vi "推導公式.vi"(3 "be":i16 min=0, 4 "al":i16 min=0, 5 "移動z":i16 min=0) -> (0 "L3":dbl, 1 "L2":dbl, 2 "L1":dbl)   [LabVIEW 2019]
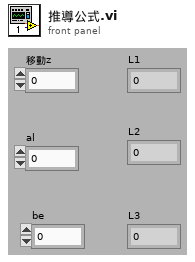
[diagram p1: front panel]
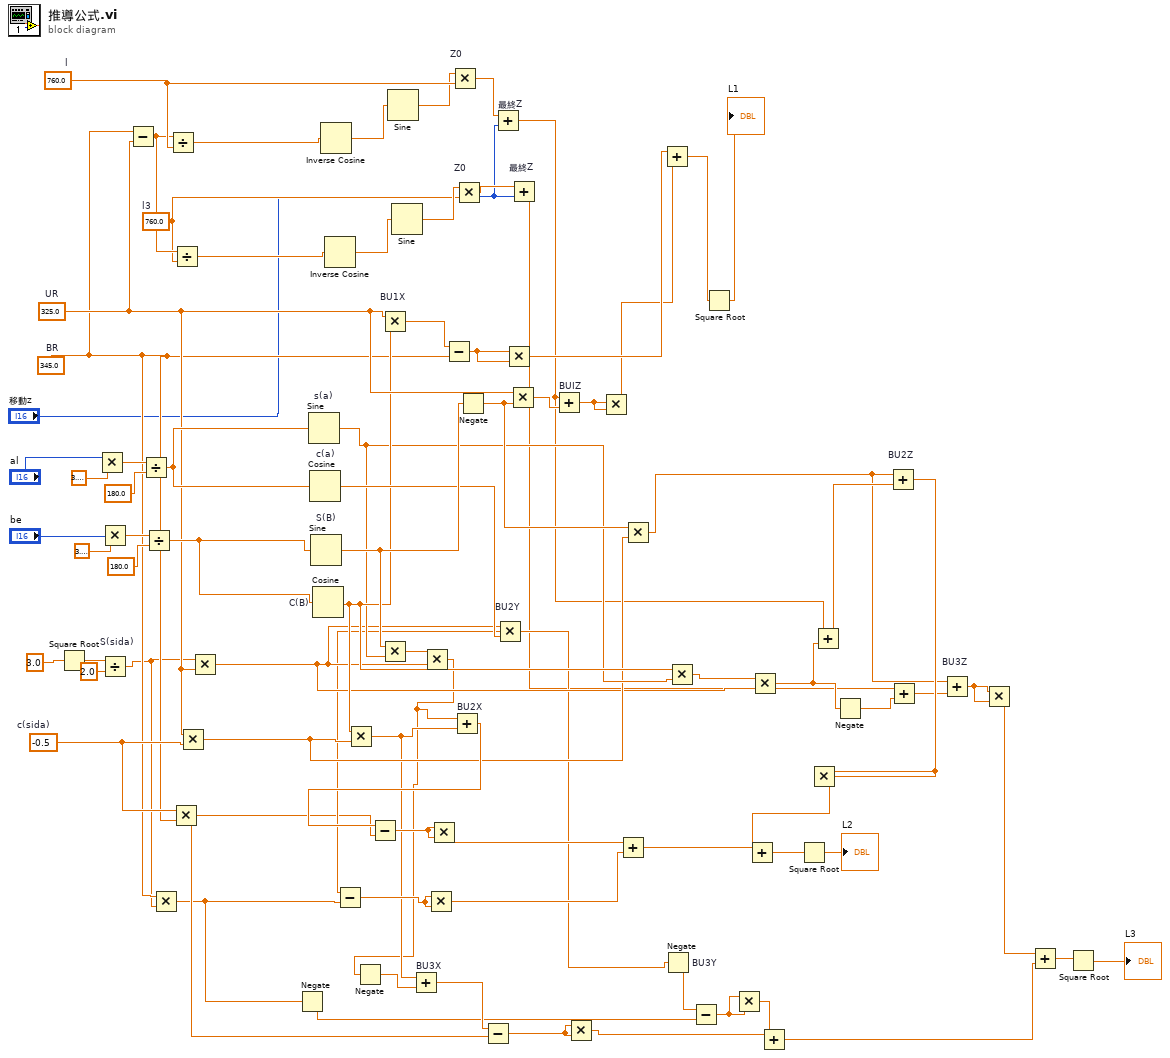
[diagram p0: block diagram]
diagram:
  w4 = 760.0  # l3
  w64 = 760.0  # l
  w29 = 345.0  # BR
  w46 = -0.5  # c(sida)
  w55 = 325.0  # UR
  n1 = Square Root(x=3.0) -> (sqrt(x)=w80:dbl)
  n2 = Multiply(x="al", y=3.141592653589793) -> (x*y=w76:dbl)
  n3 = Multiply(x="be", y=3.141592653589793) -> (x*y=w73:dbl)
  n4 = Divide "S(sida)"(x=w80, y=2.0) -> (x/y=w28:dbl)
  n5 = Subtract(x=w29, y=w55) -> (x-y=w6:dbl)
  n6 = Divide(x=w76, y=180.0) -> (x/y=w70:dbl)
  n7 = Divide(x=w73, y=180.0) -> (x/y=w69:dbl)
  n8 = Multiply(x=w29, y=w28) -> (x*y=w24:dbl)
  n9 = Divide(x=w6, y=w64) -> (x/y=w66:dbl)
  n10 = Multiply(x=w46, y=w29) -> (x*y=w25:dbl)
  n11 = Divide(x=w6, y=w4) -> (x/y=w5:dbl)
  n12 = Multiply(x=w55, y=w46) -> (x*y=w36:dbl)
  n13 = Multiply(x=w28, y=w55) -> (x*y=w34:dbl)
  n14 = Negate(x=w24) -> (-x=w22:dbl)
  n15 = Sine "s(a)"(x=w70) -> (sin(x)=w49:dbl)
  n16 = Cosine "c(a)"(x=w70) -> (cos(x)=w52:dbl)
  n17 = Sine "S(B)"(x=w69) -> (sin(x)=w54:dbl)
  n18 = Cosine "C(B)"(x=w69) -> (cos(x)=w50:dbl)
  n19 = Inverse Cosine(1:w66) -> (0:w65:dbl)
  n20 = Inverse Cosine(1:w5) -> (0:w8:dbl)
  n21 = Multiply(x=w50, y=w36) -> (x*y=w35:dbl)
  n22 = Multiply "BU1X"(x=w55, y=w50) -> (x*y=w68:dbl)
  n23 = Multiply(x=w54, y=w49) -> (x*y=w53:dbl)
  n24 = Sine(x=w65) -> (sin(x)=w63:dbl)
  n25 = Sine(x=w8) -> (sin(x)=w7:dbl)
  n26 = Multiply(x=w53, y=w34) -> (x*y=w32:dbl)
  n27 = Negate(x=w32) -> (-x=w33:dbl)
  n28 = Add "BU3X"(x=w35, y=w33) -> (x+y=w30:dbl)
  n29 = Subtract(x=w68, y=w29) -> (x-y=w67:dbl)
  n30 = Multiply "Z0"(x=w63, y=w64) -> (x*y=w62:dbl)
  n31 = Add "BU2X"(x=w32, y=w35) -> (x+y=w47:dbl)
  n32 = Subtract(x=w47, y=w25) -> (x-y=w45:dbl)
  n33 = Multiply(x=w45, y=w45) -> (x*y=w44:dbl)
  n34 = Multiply "Z0"(x=w7, y=w4) -> (x*y=w3:dbl)
  n35 = Negate(x=w54) -> (-x=w51:dbl)
  n36 = Subtract(x=w30, y=w25) -> (x-y=w27:dbl)
  n37 = Add "最終Z"(x=w62, y="移動z") -> (x+y=w16:dbl)
  n38 = Multiply "BU2Y"(x=w34, y=w52) -> (x*y=w31:dbl)
  n39 = Subtract(x=w31, y=w24) -> (x-y=w43:dbl)
  n40 = Multiply(x=w43, y=w43) -> (x*y=w42:dbl)
  n41 = Multiply(x=w67, y=w67) -> (x*y=w59:dbl)
  n42 = Multiply(x=w55, y=w51) -> (x*y=w61:dbl)
  n43 = Add "最終Z"(x=w3, y="移動z") -> (x+y=w1:dbl)
  n44 = Add "BUIZ"(x=w16, y=w61) -> (x+y=w60:dbl)
  n45 = Multiply(x=w27, y=w27) -> (x*y=w26:dbl)
  n46 = Multiply(x=w60, y=w60) -> (x*y=w58:dbl)
  n47 = Add(x=w44, y=w42) -> (x+y=w41:dbl)
  n48 = Multiply(x=w51, y=w36) -> (x*y=w14:dbl)
  n49 = Add(x=w59, y=w58) -> (x+y=w57:dbl)
  n50 = Negate "BU3Y"(x=w31) -> (-x=w23:dbl)
  n51 = Multiply(x=w50, y=w49) -> (x*y=w48:dbl)
  n52 = Subtract(x=w23, y=w22) -> (x-y=w21:dbl)
  n53 = Square Root(x=w57) -> (sqrt(x)=→"L1":dbl)
  n54 = Multiply(x=w21, y=w21) -> (x*y=w20:dbl)
  n55 = Multiply(x=w48, y=w34) -> (x*y=w18:dbl)
  n56 = Add(x=w26, y=w20) -> (x+y=w12:dbl)
  n57 = Add(x=w16, y=w18) -> (x+y=w19:dbl)
  n58 = Negate(x=w18) -> (-x=w17:dbl)
  n59 = Add "BU2Z"(x=w14, y=w19) -> (x+y=w40:dbl)
  n60 = Multiply(x=w40, y=w40) -> (x*y=w39:dbl)
  n61 = Add(x=w41, y=w39) -> (x+y=w38:dbl)
  n62 = Square Root(x=w38) -> (sqrt(x)=→"L2":dbl)
  n63 = Add(x=w1, y=w17) -> (x+y=w15:dbl)
  n64 = Add "BU3Z"(x=w14, y=w15) -> (x+y=w13:dbl)
  n65 = Multiply(x=w13, y=w13) -> (x*y=w11:dbl)
  n66 = Add(x=w11, y=w12) -> (x+y=w10:dbl)
  n67 = Square Root(x=w10) -> (sqrt(x)=→"L3":dbl)
